vi "Determine Warnings.vi"() -> ()   [LabVIEW 2014]
doc: "This VI will determine whether a temperature warning is needed based on the current, minimum, and maximum temperatures being inputted. \nInputs: Current Temp, Max Temp, Min Temp\nOutputs: Warning Text, Warning?\nEmma Gordon\n9/8/16"
panel:
  out "Warning?":bool
  out "Warning Text":string
  in  "Min Temp":dbl
  in  "Max Temp":dbl
  in  "Current Temp":dbl
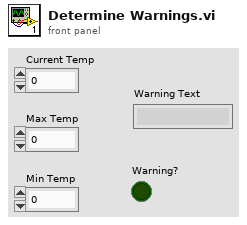
[diagram p1: front panel]
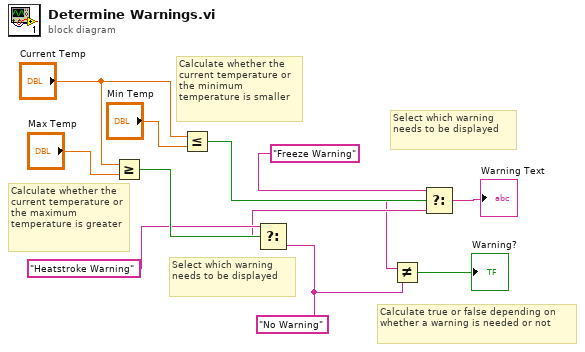
[diagram p0: block diagram]
diagram:
  w2 = "No Warning"
  # "Select which warning needs to be displayed"
  # "Calculate true or false depending on whether a warning is needed or not"
  # "Select which warning needs to be displayed"
  # "Calculate whether the current temperature or the maximum temperature is greater"
  # "Calculate whether the current temperature or the minimum temperature is smaller"
  n1 = Greater Or Equal?(x="Current Temp", y="Max Temp") -> (x >= y?=w8:bool)
  n2 = Less Or Equal?(x="Current Temp", y="Min Temp") -> (x <= y?=w6:bool)
  n3 = Select(t="Heatstroke Warning", s=w8, f=w2) -> (s? t:f=w4:string)
  n4 = Select(t="Freeze Warning", s=w6, f=w4) -> (s? t:f=w3:string)
  "Warning Text" <- w3
  n5 = Not Equal?(x=w3, y=w2) -> (x != y?=→"Warning?":bool)
